vi "uActor_Send to Self.vi"(8 "error in (no error)":errorcluster, 10 "uMsg":refnum<class "uMsg.lvclass">, 11 "uActor in":refnum<class "uActor.lvclass">) -> (0 "error out":errorcluster, 3 "uActor out":refnum<class "uActor.lvclass">)   [LabVIEW 2023, in "uFramework.lvlib" / "uActor.lvclass"]
doc: "Use by an actor to enqueue a message to self."
uses:
  uActor.lvclass
  uMsg/uMsg.lvclass
  uActor.lvclass/uActor.ctl
  uMsg/uMsg.lvclass/uMsg.ctl
  uTransport_uActor/uTransport_uActor.lvclass/uTransport_uActor.ctl
  uTransport_uActor/uTransport_uActor_SendMsg.vi
  uMsg/uMsg Update Timestamp.vi
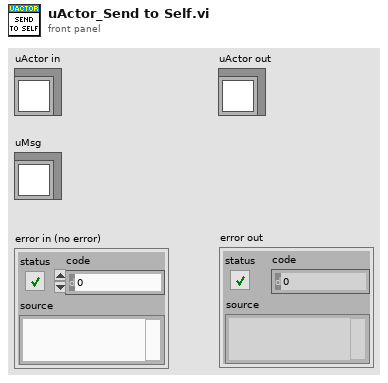
[diagram p1: front panel]
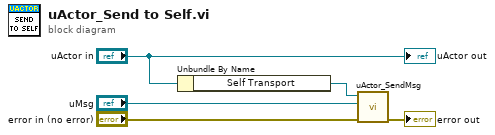
[diagram p0: block diagram]
diagram:
  n1 = Unbundle By Name("uActor in") -> ("Self Transport"=w4:refnum<class "uTransport_uActor.lvclass">)
  n2 = call "uActor_SendMsg.vi"("error in (no error)"="error in (no error)", "Msg"="uMsg", "uActor Transport"=w4) -> ("error out"=→"error out":errorcluster)  [unwired: 8 in]
  "uActor out" <- "uActor in"
